vi "StartMeasurement.vi"(8 "error in (no error)":errorcluster, 9 "Variant":variant, 10 "Option":i32, 11 "Avantes in":refnum<class "Avantes.lvclass">) -> (0 "error out":errorcluster, 3 "Avantes out":refnum<class "Avantes.lvclass">)   [LabVIEW 2018, in "Avantes.lvclass"]
uses:
  <instrlib>/Classes/CCD/Avantes/Avantes.lvclass
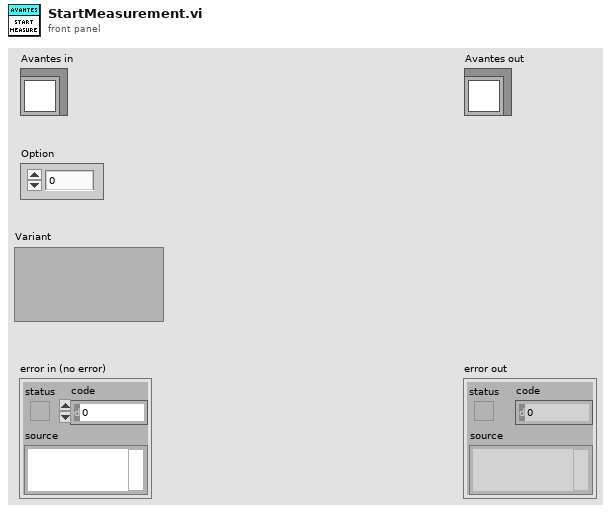
[diagram p1: front panel]
types:
  T1 = cluster{"Frames":i32, "Start Pixel":u16, "Stop Pixel":u16}
  T2 = typedef "clusterdef.ctl" = cluster{"Len":u16, "ConfigVersion":u16, "UserFriendlyId":u8[], "DetectorType":cluster{"SensorType":u8, "NrPixels":u16, "Fit":sgl[], "NLEnable":u8, "NLCorrect":dbl[], "LowNLCounts":dbl, "HighNLCounts":dbl, "Gain":sgl[], "Reserved":sgl, "Offset":sgl[], "Extern Offset":sgl, "DefectivePixels":u16[]}, "IrradianceType":cluster{"SpectrumCalibrationType":cluster{"SmoothingType":cluster{"m_SmoothPix":u16, "SmoothModel":u8}, "CalInttime":sgl, "CalibConvers":sgl[]}, "CalibrationType":u8, "FiberDiameter":i32}, "SpectrumCalibrationType":cluster{"SmoothingType":cluster{"m_SmoothPix":u16, "SmoothModel":u8}, "CalInttime":sgl, "CalibConvers":sgl[]}, "SpectrumCorrectionType":sgl[], "StandAloneType":cluster{"StandAloneType":u8, "MeasConfigType":cluster{"StartPixel":u16, "StopPixel":u16, "IntegrationTime":sgl, "IntegrationDelay":u32, "NrAverages":u32, "DarkCorrectionType":cluster{"Enable CorDynDark":u8, "ForgetPercentage":u8}, "SmoothingType":cluster{"SmoothPix":u16, "SmoothModel":u8}, "SatDetection":u8, "TriggerType":cluster{"Trigger Mode":u8, "Trigger Source":u8, "Trigger SourceType":u8}, "ControlSettingsType":cluster{"StrobeControl":u16, "LaserDelay":u32, "LaserWidth":u32, "LaserWaveLength":sgl, "StoreToRam":u16}}, "Nmsr":i16}, "DynamicStorageType":cluster{"Nmsr":i32, "Reserved":u8[]}, "TempSensorType":sgl[], "TecControlType":cluster{"Enable":u8, "Setpoint":sgl, "Fit[NR_DAC_POL_COEF]":sgl[]}, "ProcessControlType":cluster{"AnalogLow":sgl[], "AnalogHigh":sgl[], "DigitalLow":sgl[], "DigitalHigh":sgl[]}, "EthernetSettingsType":cluster{"IpAddr":u32, "NetMask":u32, "Gateway":u32, "DhcpEnabled":u8, "TcpPort":u16, "LinkStatus":u8}, "Reserved":u8[], "OemData":u8[]}
  T3 = cluster{"StartPixel":u16, "StopPixel":u16, "IntegrationTime":sgl, "IntegrationDelay":u32, "NrAverages":u32, "DarkCorrectionType":cluster{"Enable CorDynDark":u8, "ForgetPercentage":u8}, "SmoothingType":cluster{"SmoothPix":u16, "SmoothModel":u8}, "SatDetection":u8, "TriggerType":cluster{"Trigger Mode":u8, "Trigger Source":u8, "Trigger SourceType":u8}, "ControlSettingsType":cluster{"StrobeControl":u16, "LaserDelay":u32, "LaserWidth":u32, "LaserWaveLength":sgl, "StoreToRam":u16}}
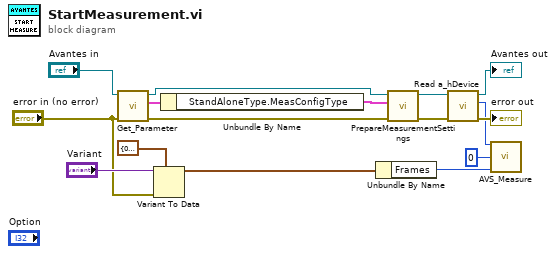
[diagram p0: block diagram]
diagram:
  n1 = call-dynamic "Get_Parameter.vi"("error in (no error)"="error in (no error)", "Avantes in"="Avantes in") -> ("error out"=w5:errorcluster, "DeviceConfig"=w14:T2, "Avantes out"=w13:refnum<class "Avantes.lvclass">)  [unwired: 7 in]
  n2 = Variant To Data(error in="error in (no error)", type=T1 {"Frames"=0, "Start Pixel"=0, "Stop Pixel"=0}, Variant="Variant") -> (data=w9:T1)  [unwired: 1 out]
  n3 = Unbundle By Name(w14) -> ("StandAloneType.MeasConfigType"=w12:T3)
  n4 = Unbundle By Name(w9) -> ("Frames"=w8:i32)
  n5 = call-dynamic "PrepareMeasurementSettings.vi"("error in (no error)"=w5, "MeasConfigType"=w12, "Avantes in"=w13) -> ("error out"=w6:errorcluster, "Avantes out"=w7:refnum<class "Avantes.lvclass">)  [unwired: 7 in]
  n6 = call-dynamic "Read a_hDevice.vi"("error in (no error)"=w6, "Avantes in"=w7) -> ("error out"=→"error out":errorcluster, "a_hDevice"=w2:i32, "Avantes out"=→"Avantes out":refnum<class "Avantes.lvclass">)  [unwired: 7 in]
  n7 = call <instrlib>:"AVS_Measure.vi"("a_hDevice"=w2, "a_hWnd"=0, "a_Nmsr"=w8) -> ()  [unwired: 12 in, 1 out]
